vi "InitialSine6221.vi"(6 "DC Offset In (A)":dbl, 8 "error in (no error)":errorcluster, 9 "Amplitude In (A)":dbl, 10 "Frequency In (Hz)":dbl, 11 "VISA Refnum in":refnum<visa-resource-name>) -> (0 "error out":errorcluster, 3 "VISA Refnum out":refnum<visa-resource-name>)   [LabVIEW 2012]
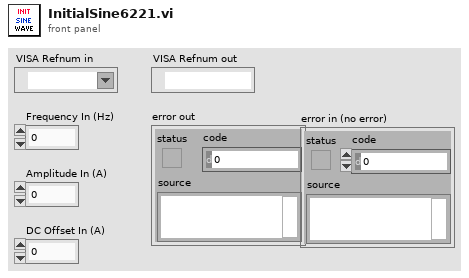
[diagram p1: front panel]
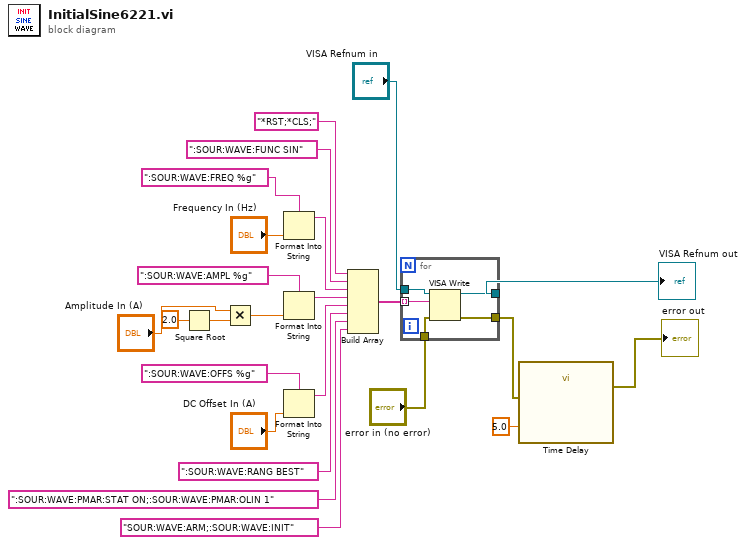
[diagram p0: block diagram]
diagram:
  n1 = Square Root(x=2.0 ("y")) -> (sqrt(x)=w24:dbl)
  n2 = Multiply(x="Amplitude In (A)", y=w24) -> (x*y=w22:dbl)
  n3 = Format Into String(format string=":SOUR:WAVE:FREQ %g", "Frequency In (Hz)") -> (resulting string=w7:string)  [unwired: 2 in, 1 out]
  n4 = Format Into String(format string=":SOUR:WAVE:AMPL %g", w22) -> (resulting string=w8:string)  [unwired: 2 in, 1 out]
  n5 = Format Into String(format string=":SOUR:WAVE:OFFS %g", "DC Offset In (A)") -> (resulting string=w9:string)  [unwired: 2 in, 1 out]
  n6 = Build Array("*RST;*CLS;" ("write buffer"), ":SOUR:WAVE:FUNC SIN" ("format string"), w7, w8, w9, ":SOUR:WAVE:RANG BEST" ("format string"), ":SOUR:WAVE:PMAR:STAT ON;:SOUR:WAVE:PMAR:OLIN 1", "SOUR:WAVE:ARM;:SOUR:WAVE:INIT" ("write buffer")) -> (w10:string[])
  n7 = for {
    tunnel: w10 -> [w29] mode=indexing
    tunnel: "VISA Refnum in" -> [w28]
    tunnel: [w27] -> w20
    tunnel: [w26] -> w4
    tunnel: "error in (no error)" -> [w25]
    n8 = VISA Write(VISA resource name=w28, write buffer=w29, error in (no error)=w25) -> (VISA resource name out=w27:refnum<visa-resource-name>, error out=w26:errorcluster)  [unwired: 1 out]
  }
  "VISA Refnum out" <- w20
  n9 = call "Time Delay"("error in (no error)"=w4, "Delay Time (s)"=5.0) -> ("error out"=→"error out":errorcluster)  [unwired: 9 in]
